vi "Core gRPC Server.vi"(8 "error in (no error)":errorcluster, 11 "CIFTemplateNode in":refnum<class "CIFCorePlugin.lvclass">) -> (0 "error out":errorcluster, 3 "CIFTemplateNode out":refnum<class "CIFCorePlugin.lvclass">)   [LabVIEW 2021, in "CIFCorePlugin.lvclass"]
uses:
  CIFCorePlugin.lvclass
  CIFCorePlugin.lvclass/CIFCorePlugin.ctl
  Grpc/CIFCorePlugin_server/RPC Service/PluginCore/PluginCore.lvclass
  Grpc/CIFCoreWrapper/CIFCoreWrapper.lvlib
  Grpc/CIFCorePlugin_client/RPC Messages/cif_common_Version.ctl
  Grpc/CIFCorePlugin_client/CIFCorePlugin_client.lvlib
  <vilib>/addons/_JKI.lib/Serialization/JSON/JKI JSON Serialization.lvlib
  Grpc/CIFCorePlugin_server/RPC Messages/cif_plugincore_Configuration.ctl
  Grpc/CIFCorePlugin_server/CIFCorePlugin_server.lvlib
  Grpc/CIFCorePlugin_server/RPC Messages/cif_plugincore_TimingOverrides.ctl
  Grpc/CIFCorePlugin_server/RPC Messages/cif_plugincore_PluginOverrides.ctl
  <vilib>/gRPC/LabVIEW gRPC Servicer/Servicer/Servicer.lvclass
  Common/CIFCoreCommon.lvlib
  Common/Typedef/Errors.ctl
  CIFUtilities/CIFLogs/CIFLogs.lvlib
  CIFUtilities/CIFLogs/Typedef/Plugin State Commands.ctl
  Grpc/CIFCoreChannel_server/RPC Service/ChannelCore/ChannelCore.lvclass
  Grpc/CIFCorePlugin_client/RPC Messages/cif_common_Status.ctl
  Grpc/CIFCoreChannel_server/RPC Messages/cif_channelcore_ChannelDirection.ctl
  Grpc/CIFCoreChannel_server/CIFCoreChannel_server.lvlib
  Grpc/CIFCoreChannel_server/RPC Messages/cif_channelcore_Channel.ctl
  Grpc/CIFCoreChannel_server/RPC Messages/cif_channelcore_Channels.ctl
  Grpc/CIFCorePlugin_client/RPC Messages/cif_common_PluginNames.ctl
  Common/Typedef/Channel Connection Data.ctl
  Common/Typedef/Channel Force Data.ctl
  Grpc/CIFCoreChannel_server/RPC Messages/cif_common_Status.ctl
  Grpc/CIFCoreChannel_server/RPC Messages/cif_channelcore_FIFOReference.ctl
  <vilib>/CIF Foundation/CIF Channels Core/ChannelCommon/typedef/New FIFO Instance Configuration.ctl
  <vilib>/CIF Foundation/CIF Channels Core/ChannelCommon/ChannelCommon.lvlib
  Common/Typedef/FIFO Publisher.ctl
  Channels/CIFChannelMng/CIFChannelMng.lvclass
  Grpc/CIFCoreChannel_server/RPC Messages/cif_channelcore_ChannelPattern.ctl
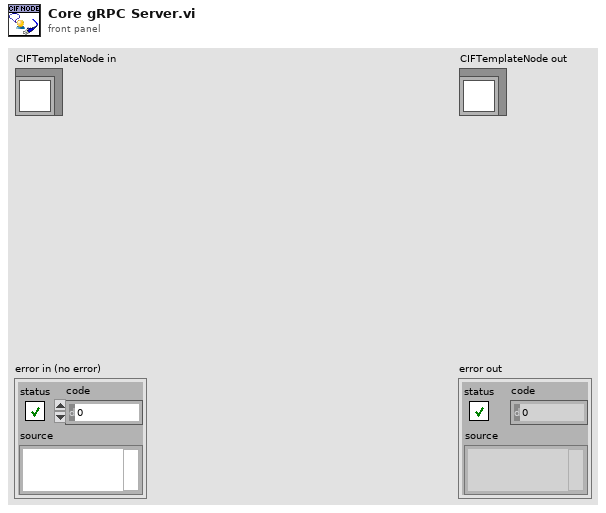
[diagram p1: front panel]
types:
  T1 = typedef "CIFCorePlugin_client.lvlib/cif_common_Status.ctl" = cluster{"code":i32, "message":string}
  T2 = typedef "CIFCorePlugin_client.lvlib/cif_common_PluginNames.ctl" = cluster{"plugin_name":string, "plugin_type":string}
  T3 = typedef "CIFCoreCommon.lvlib/Errors.ctl" = enum16{"Invalid Clock ID", "Long Sleep", "gRPC Server Not Found", "Config Parse", "Timestamp Wrap", "Delayed Execution", "Duplicate Channel", "Missing Channel", "Incorrect Type", "Flatten Error", "Unflatten Data", "Unique Name", "Plugin Not Found", "Plugin Type Not Found", "Plugin Version Not Found", "Manager Not Found", "Numerical Issue", "Time Jump", "Clock ID Match", "Channel Length", "Plugin Connection", "gRPC Server Connection", "PPL Name Match", "Build", "Config Log Parse", "Plugin Load", "UI Subpanel Load", "Python Name", "Invalid Name", "Unable to Change Ch Buffer"}
  T4 = typedef "CIFCorePlugin_client.lvlib/cif_common_Version.ctl" = cluster{"major":u32, "minor":u32, "fix":u32, "build":u32}
  T5 = typedef "CIFCorePlugin_server.lvlib/cif_plugincore_Configuration.ctl" = cluster{"json_config":string}
  T6 = typedef "CIFCorePlugin_server.lvlib/cif_plugincore_PluginOverrides.ctl" = cluster{"timing_overrides":T7}
  T7 = typedef "CIFCorePlugin_server.lvlib/cif_plugincore_TimingOverrides.ctl" = cluster{"override_timing":bool, "skip_sleep":bool, "period":dbl}
  T8 = typedef "CIFCoreCommon.lvlib/Channel Connection Data.ctl" = cluster{"Publisher Name":string, "Subscriber Name":string, "Connection Data":u8[]}
  T9 = typedef "CIFCoreCommon.lvlib/Channel Force Data.ctl" = cluster{"Channel Name":string, "Force Data":u8[], "Force Active":bool}
  T10 = typedef "CIFCoreCommon.lvlib/FIFO Publisher.ctl" = cluster{"Publisher Name":string, "New FIFO Instance Config":T11}
  T11 = typedef "ChannelCommon.lvlib/New FIFO Instance Configuration.ctl" = cluster{"Backpressure":bool, "Bytes/Message Override":u32, "Messages/FIFO Override":u32, "Custom Data":u8[]}
  T12 = typedef "CIFCoreChannel_server.lvlib/cif_channelcore_FIFOReference.ctl" = cluster{"publisher_instance_name":string, "custom_connect":u8[], "status":T13}
  T13 = typedef "CIFCoreChannel_server.lvlib/cif_common_Status.ctl" = cluster{"code":i32, "message":string}
  T14 = typedef "CIFCoreChannel_server.lvlib/cif_channelcore_Channels.ctl" = cluster{"channels":T15[]}
  T15 = typedef "CIFCoreChannel_server.lvlib/cif_channelcore_Channel.ctl" = cluster{"name":string, "direction":T16, "type":string, "custom_config":u8[], "connected":bool, "connected_name":string, "forced":bool, "channel_pattern":T17}
  T16 = typedef "CIFCoreChannel_server.lvlib/cif_channelcore_ChannelDirection.ctl" = enum32{"CHANNELDIRECTION_UNKNOWN", "CHANNELDIRECTION_PUBLISHER", "CHANNELDIRECTION_SUBSCRIBER"}
  T17 = typedef "CIFCoreChannel_server.lvlib/cif_channelcore_ChannelPattern.ctl" = enum32{"CHANNELPATTERN_UNKNOWN", "CHANNELPATTERN_TAG", "CHANNELPATTERN_FIFO", "CHANNELPATTERN_MULTIFIFO", "CHANNELPATTERN_BACKPRESSUREFIFO"}
  T18 = typedef "grpc-lvsupport-release.lvlib/grpcId.ctl" = u64
  T19 = typedef "CIFLogs.lvlib/Plugin State Commands.ctl" = enum16{"Create", "Configure", "Run", "Pause", "Destroy", "Connect", "Force", "FIFO Instance"}
  T20 = typedef "CIFCoreCommon.lvlib/Plugin Status.ctl" = cluster{"State":T21, "Timing Statistics (us)":T22, "FIFO Statistics (us)":T24, "error":T25, "Monitor Doubles":T26, "Monitor U64":T27, "Monitor I64":T28}
  T21 = typedef "CIFCoreCommon.lvlib/Plugin State.ctl" = enum32{"Null", "Creating", "Listening", "Running", "CleaningUp", "Destroying"}
  T22 = typedef "CIFCoreCommon.lvlib/Timing Statistics.ctl" = cluster{"Period":T23, "Wake Error":T23, "Execute":T23, "Housekeep":T23, "Idle":T23, "Cleanup":T23, "Custom 1":T23, "Custom 2":T23}
  T23 = typedef "CIFCoreCommon.lvlib/Timing Stats Base.ctl" = cluster{"Max":i64, "Avg":dbl, "Min":i64}
  T24 = typedef "CIFCoreCommon.lvlib/FIFO Statistics.ctl" = cluster{"From T0":T23, "From Previous Plugin":T23, "Output Error":T23}
  T25 = typedef "CIFCoreCommon.lvlib/Simple Error.ctl" = cluster{"status":bool, "code":i32}
  T26 = typedef "CIFCoreCommon.lvlib/Monitor Doubles.ctl" = cluster{"1":dbl, "2":dbl, "3":dbl, "4":dbl}
  T27 = typedef "CIFCoreCommon.lvlib/Monitor U64.ctl" = cluster{"1":u64, "2":u64, "3":u64, "4":u64}
  T28 = typedef "CIFCoreCommon.lvlib/Monitor I64.ctl" = cluster{"1":i64, "2":i64, "3":i64, "4":i64}
  T29 = typedef "CIFCorePlugin_client.lvlib/cif_plugincore_StatusData.ctl" = cluster{"state":T30, "timing_statistics":T31, "fifo_statistics":T33, "error":T34, "monitor_doubles":T35, "monitor_u64s":T36, "monitor_i64s":T37}
  T30 = typedef "CIFCorePlugin_client.lvlib/cif_plugincore_StatusData_PluginState.ctl" = enum32{"PLUGINSTATE_UNKNOWN", "PLUGINSTATE_CREATING", "PLUGINSTATE_LISTENING", "PLUGINSTATE_RUNNING", "PLUGINSTATE_CLEANINGUP", "PLUGINSTATE_DESTROYING"}
  T31 = typedef "CIFCorePlugin_client.lvlib/cif_plugincore_TimingStatistics.ctl" = cluster{"period":T32, "wake_error":T32, "execute":T32, "housekeep":T32, "idle":T32, "cleanup":T32, "custom_1":T32, "custom_2":T32}
  T32 = typedef "CIFCorePlugin_client.lvlib/cif_common_TimingStats.ctl" = cluster{"max":i64, "min":i64, "avg":dbl}
  T33 = typedef "CIFCorePlugin_client.lvlib/cif_plugincore_FifoStatistics.ctl" = cluster{"from_t0":T32, "from_previous_plugin":T32, "output_error":T32}
  T34 = typedef "CIFCorePlugin_client.lvlib/cif_plugincore_Error.ctl" = cluster{"status":bool, "code":i32}
  T35 = typedef "CIFCorePlugin_client.lvlib/cif_plugincore_MonitorDoubles.ctl" = cluster{"double_1":dbl, "double_2":dbl, "double_3":dbl, "double_4":dbl}
  T36 = typedef "CIFCorePlugin_client.lvlib/cif_plugincore_MonitorU64.ctl" = cluster{"u64_1":u64, "u64_2":u64, "u64_3":u64, "u64_4":u64}
  T37 = typedef "CIFCorePlugin_client.lvlib/cif_plugincore_MonitorI64.ctl" = cluster{"i64_1":i64, "i64_2":i64, "i64_3":i64, "i64_4":i64}
  T38 = typedef "CIFCoreCommon.lvlib/Version.ctl" = cluster{"Major":i32, "Minor":i32, "Fix":i32, "Build":i32}
  T39 = typedef "CIFCoreChannel_server.lvlib/cif_channelcore_ConnectSubscriber.ctl" = cluster{"subscriber_name":string, "publisher_name":string, "custom_connect":u8[]}
  T40 = typedef "CIFCoreChannel_server.lvlib/cif_channelcore_ForceChannel.ctl" = cluster{"channel_name":string, "force":bool, "force_data":u8[]}
  T41 = typedef "CIFCoreChannel_server.lvlib/cif_channelcore_FIFOInstance.ctl" = cluster{"publisher_name":string, "retry_on_timeout":bool, "bytes_per_message_override":u32, "message_per_fifo_override":u32, "custom_data":u8[]}
  T42 = typedef "CIFChannelMng.lvclass/FIFO Publisher Return.ctl" = cluster{"FIFO Instance Config":T43, "error":errorcluster, "Added":bool}
  T43 = typedef "ChannelCommon.lvlib/New FIFO Instance Response.ctl" = cluster{"Publisher":string, "Custom Data":u8[]}
  T44 = typedef "CIFCoreChannel_server.lvlib/cif_channelcore_FIFOInstanceName.ctl" = cluster{"publisher_instance_name":string}
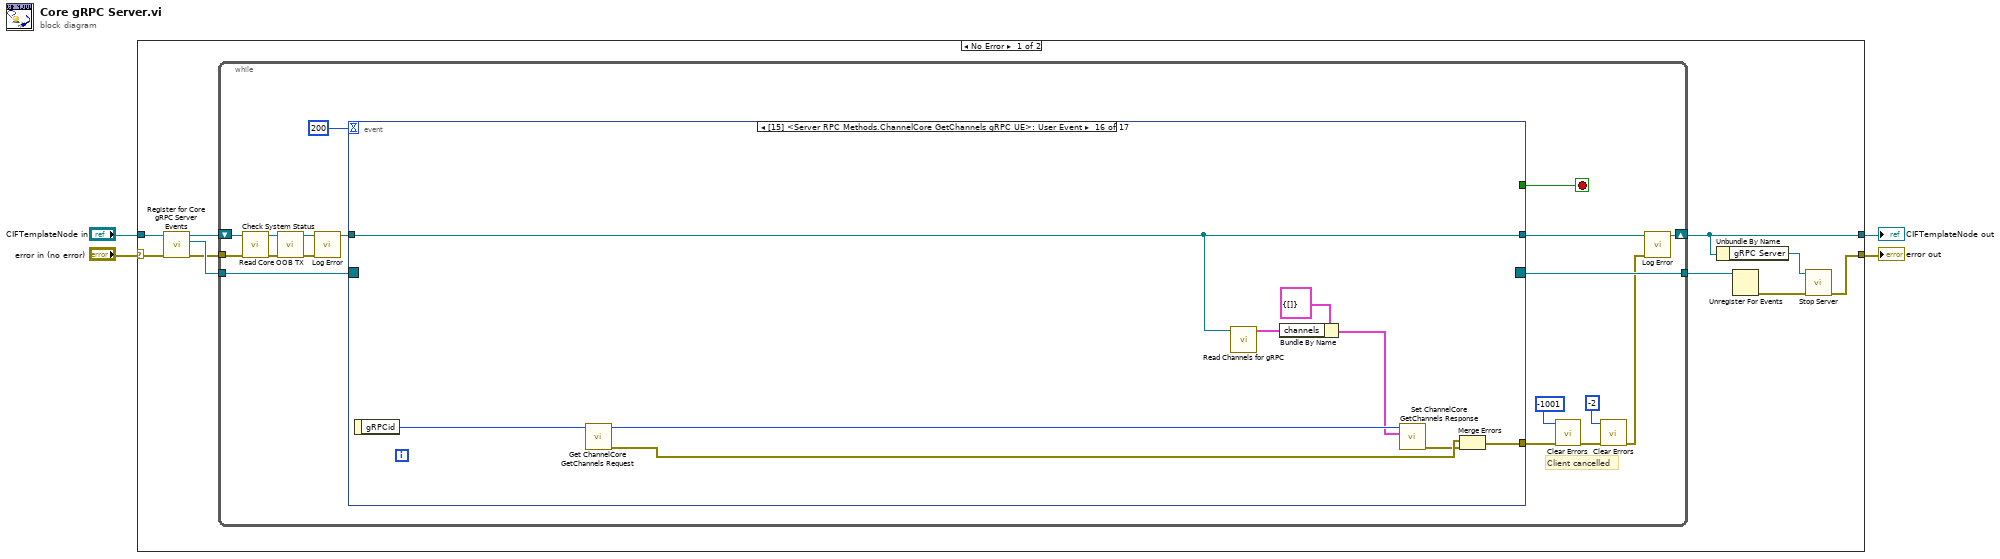
[diagram p0: block diagram]
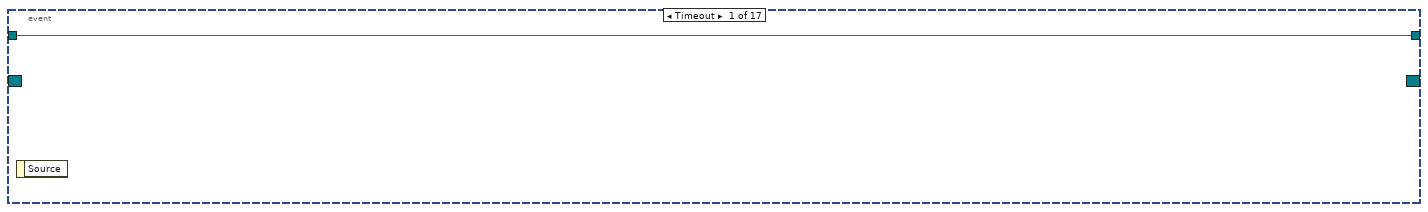
[diagram p2: hidden frame]
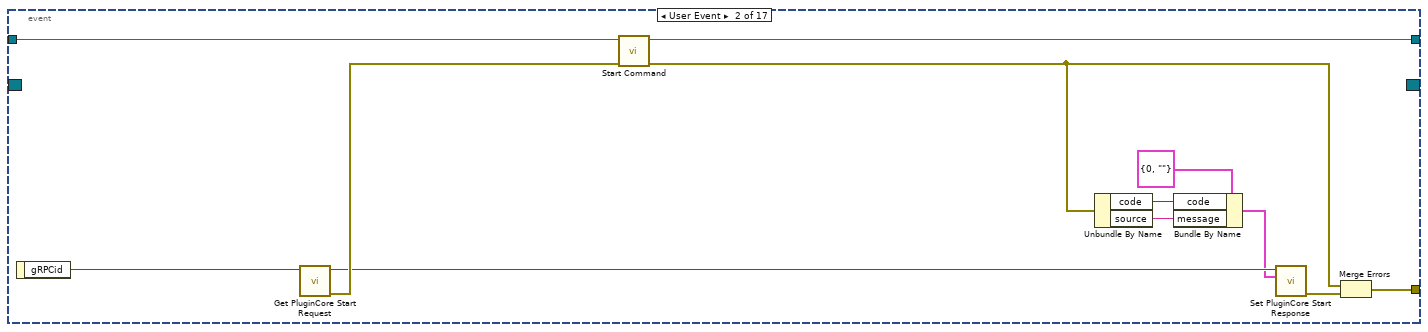
[diagram p3: hidden frame]
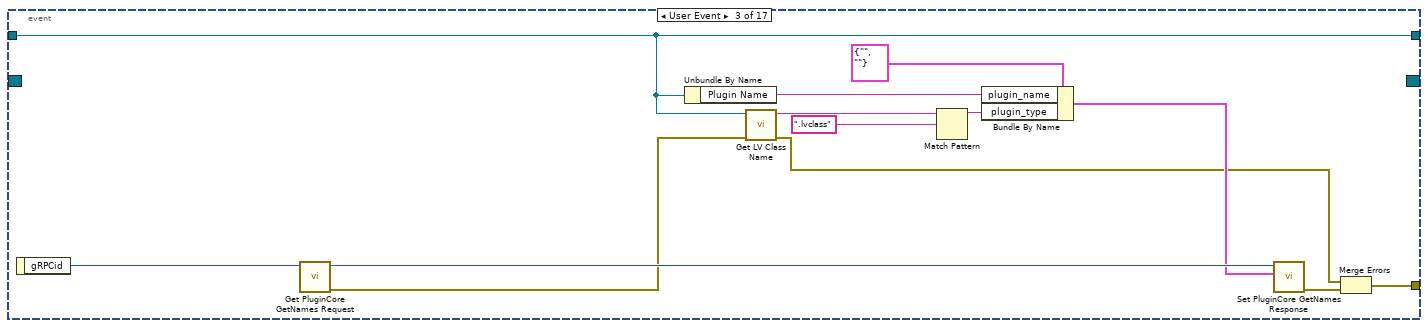
[diagram p4: hidden frame]
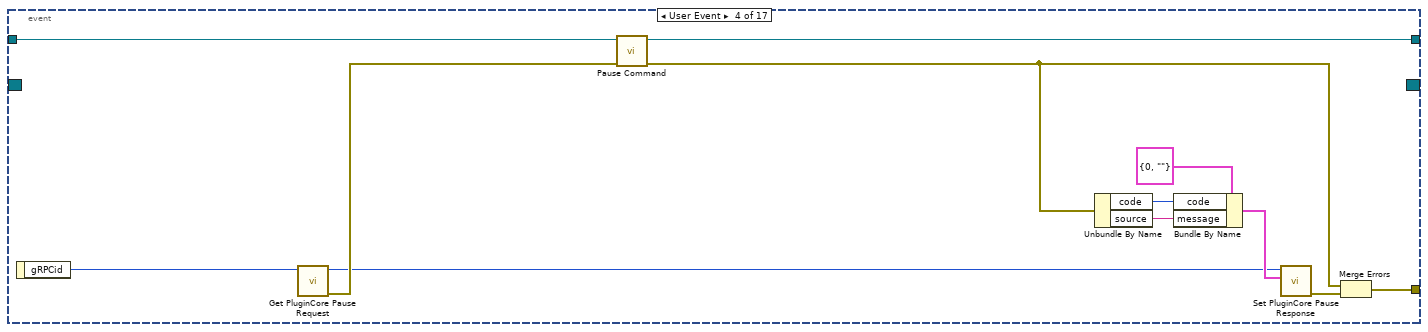
[diagram p5: hidden frame]
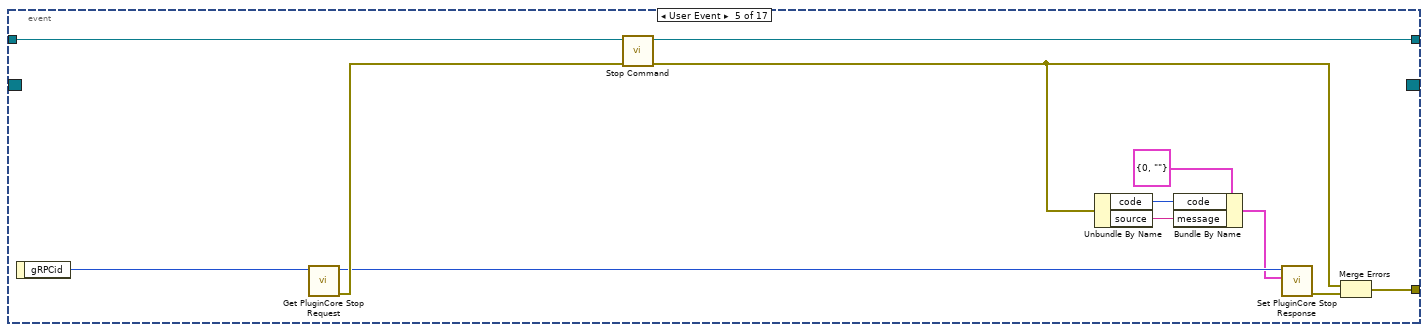
[diagram p6: hidden frame]
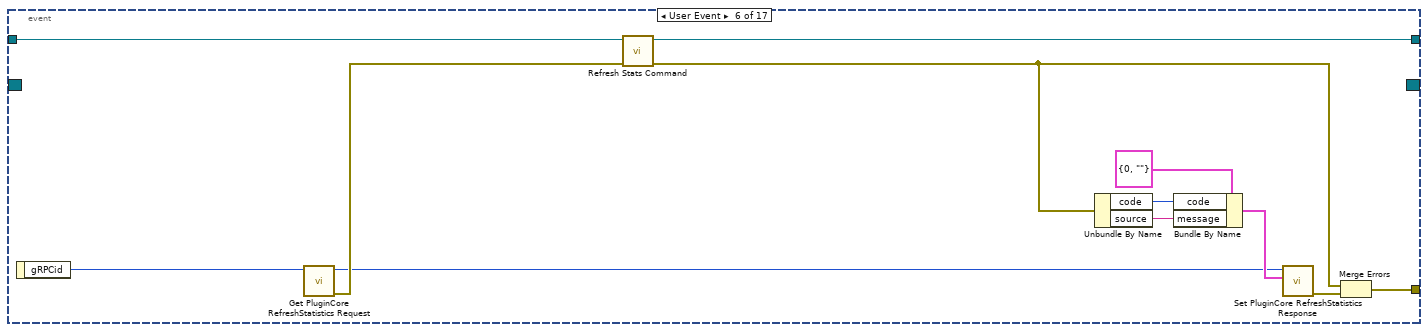
[diagram p7: hidden frame]
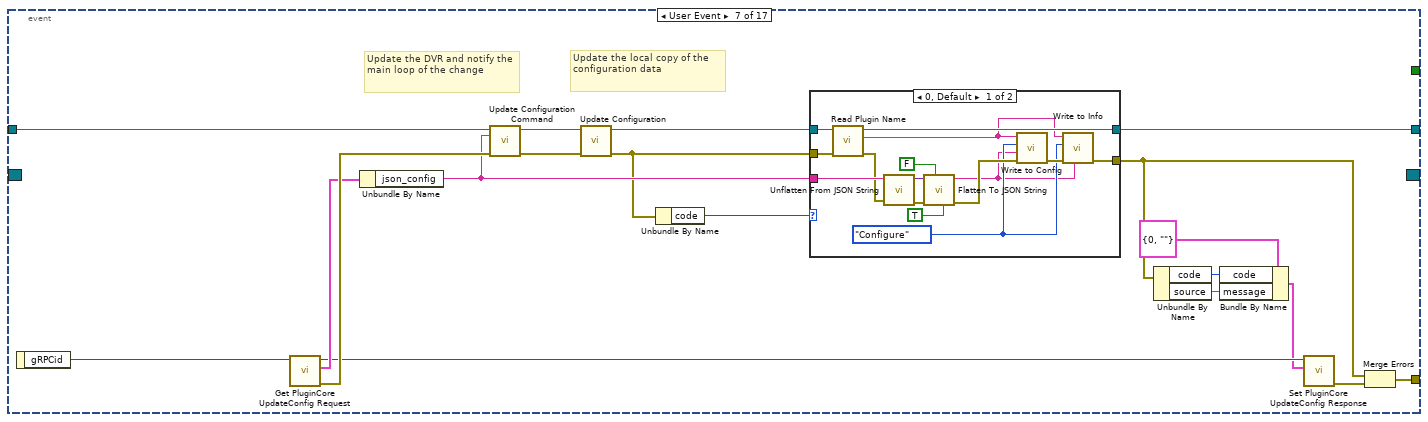
[diagram p8: hidden frame]
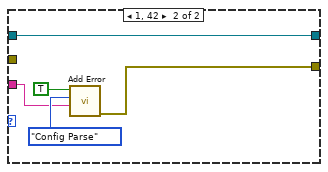
[diagram p9: hidden frame]
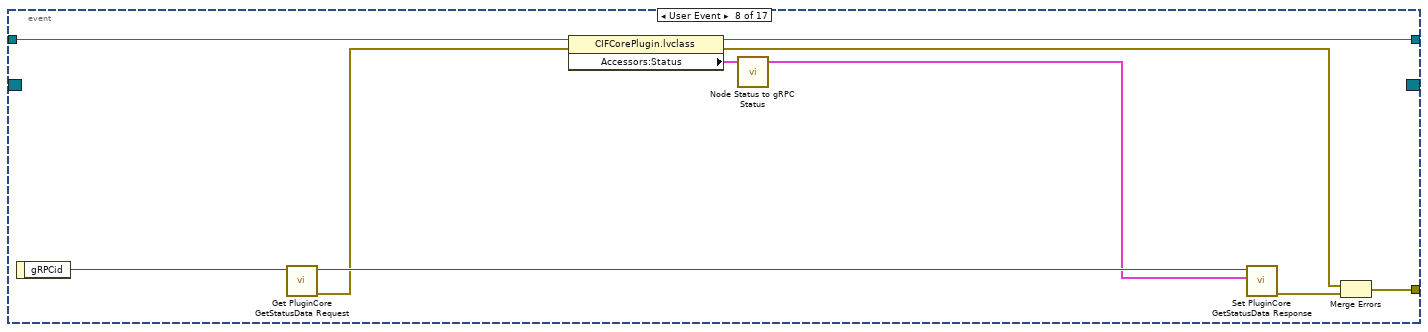
[diagram p10: hidden frame]
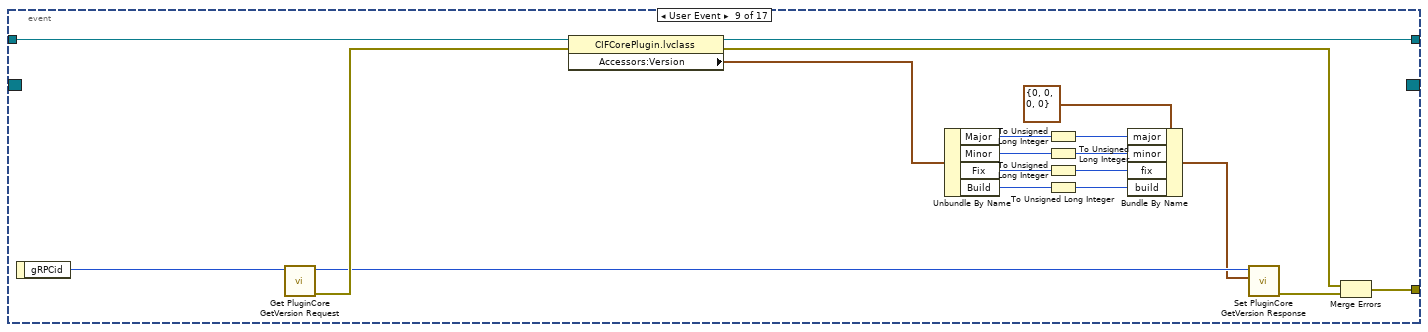
[diagram p11: hidden frame]
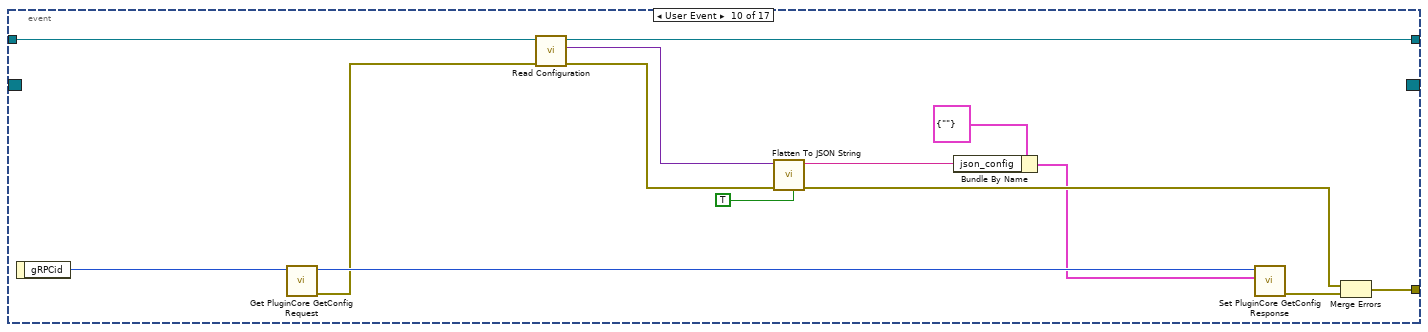
[diagram p12: hidden frame]
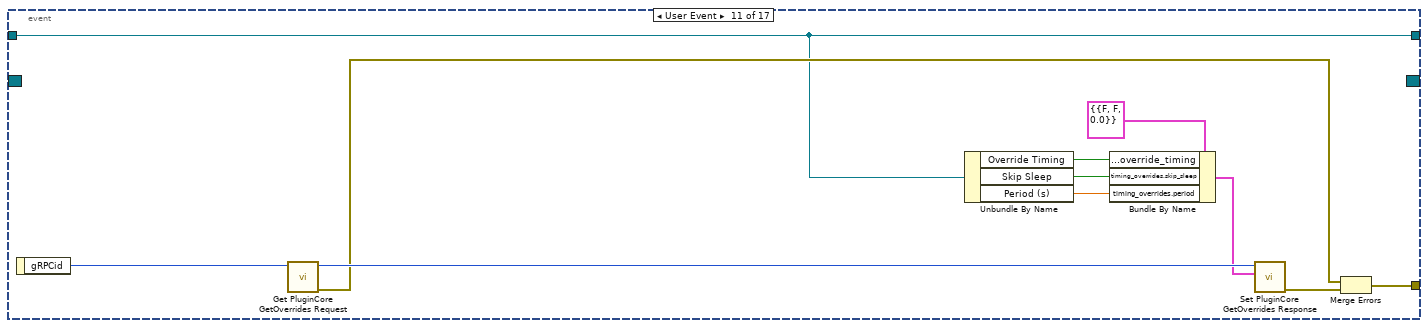
[diagram p13: hidden frame]
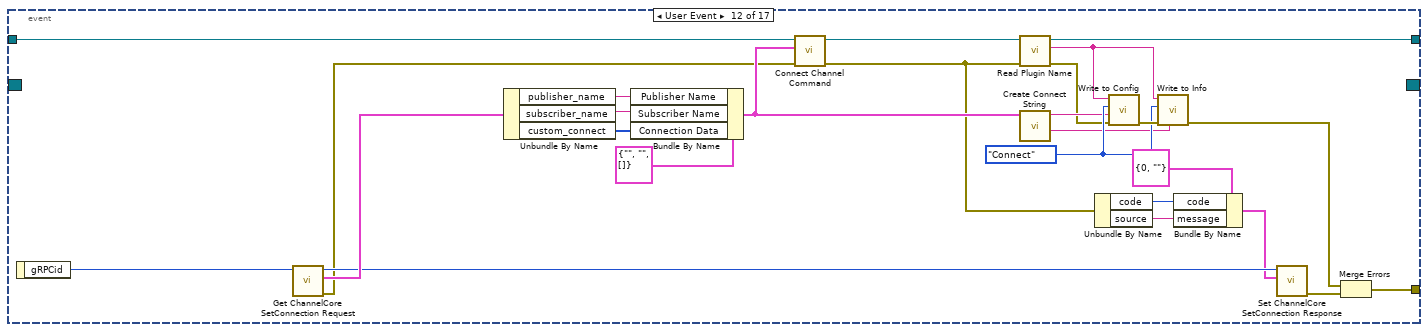
[diagram p14: hidden frame]
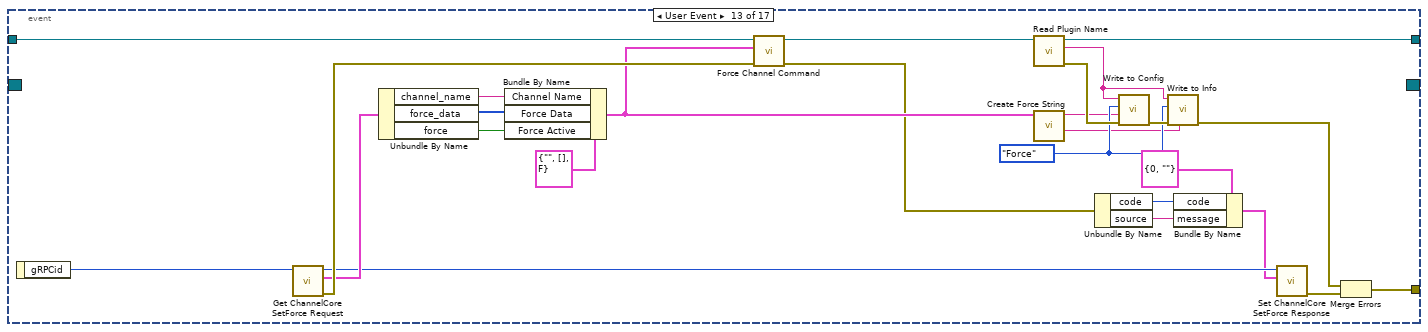
[diagram p15: hidden frame]
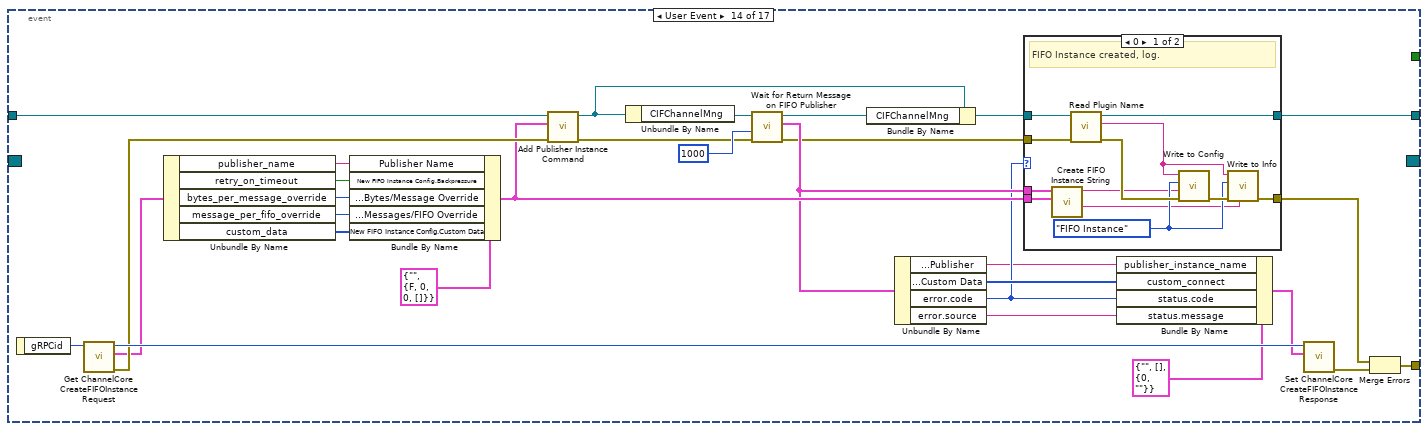
[diagram p16: hidden frame]
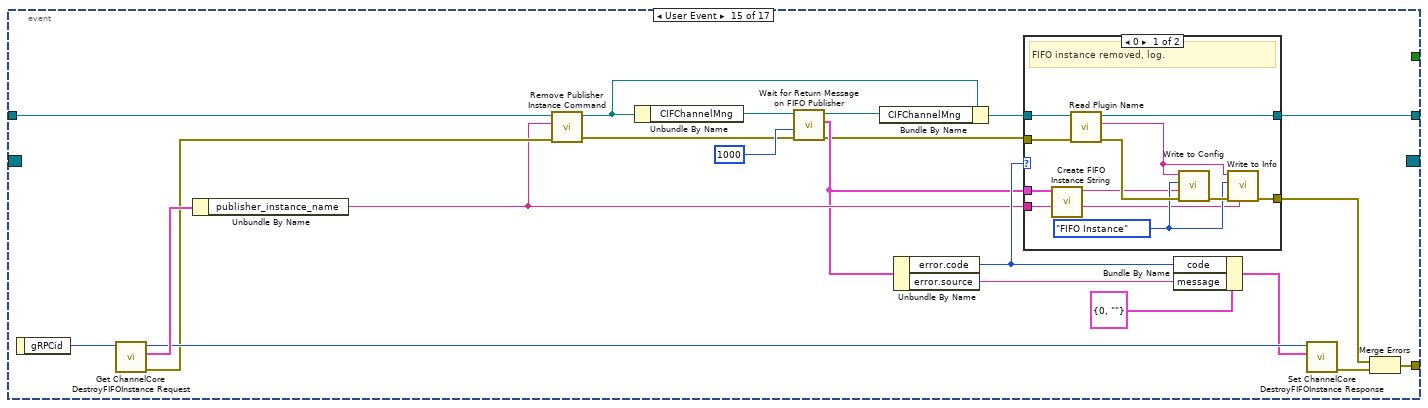
[diagram p18: hidden frame]
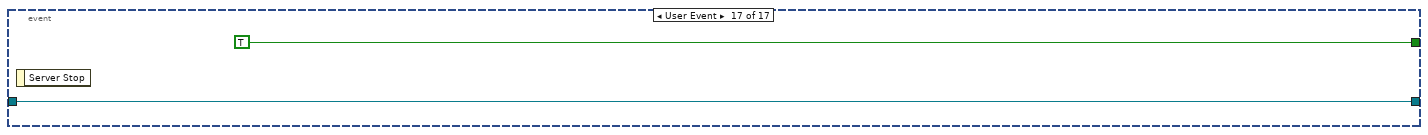
[diagram p20: hidden frame]
diagram:
  n1 = case shown="No Error" "error in (no error)" {
    selector: "error in (no error)" -> [w13 w331]
    tunnel: "CIFTemplateNode in" -> [w14 w332]
    tunnel: [w8 w332] -> w2
    tunnel: [w5 w331] -> w1
    frame No Error {
      n2 = call "Register for Core gRPC Server Events.vi"("error in (no error)"=w13, "CIFCorePlugin in"=w14) -> ("error out"=w11:errorcluster, "Event Registration Refnum"=w12:refnum<event-registration>, "CIFCorePlugin out"=w10:refnum<class "CIFCorePlugin.lvclass">)  [unwired: 7 in]
      n3 = while {
        tunnel: w12 -> [w32]
        tunnel: w11 -> [w23]
        tunnel: [w29] -> w9
        shift-right: [w27] -> w8
        shift-left: w10 -> [w22]
        stop <- w30 stop-if-true
        # "Client cancelled"
        n4 = call "Check System Status.vi"("error in (no error)"=w23, "CIFCorePlugin in"=w22) -> ("error out"=w21:errorcluster, "CIFCorePlugin out"=w20:refnum<class "CIFCorePlugin.lvclass">)  [unwired: 8 in]
        n5 = call "Read Core OOB TX.vi"("error in (no error)"=w21, "CIFCorePlugin in"=w20) -> ("error out"=w24:errorcluster, "CIFCorePlugin out"=w26:refnum<class "CIFCorePlugin.lvclass">)  [unwired: 8 in]
        n6 = call "Log Error.vi"("error in (no error)"=w24, "CIFCorePlugin in"=w26) -> ("CIFCorePlugin out"=w25:refnum<class "CIFCorePlugin.lvclass">)  [unwired: 8 in, 1 out]
        n7 = event shown="[15] <Server RPC Methods.ChannelCore GetChannels gRPC UE>: User Event" {
          selector: w32 -> [_ _ _ _ _ _ _ _ _ _ _ _ _ _ _ _ _]
          dyn-events: [_ _ _ _ _ _ _ _ _ _ _ _ _ _ _ _ _] -> w29
          timeout: 200 -> [_ _ _ _ _ _ _ _ _ _ _ _ _ _ _ _ _]
          tunnel: w25 -> [w33 w36 w52 w61 w73 w85 w100 w135 w161 w167 w180 w190 w215 w242 w287 w320 w329]
          tunnel: [_ w38 w57 w67 w79 w91 w113 w143 w162 w176 w187 w211 w237 w268 w304 w328 _] -> w18
          tunnel: [w33 w35 w52 w60 w72 w84 w101 w141 w160 w164 w180 w192 w218 w264 w303 w320 w329] -> w28
          tunnel: [_ _ _ _ _ _ _ _ _ _ _ _ _ _ _ _ TRUE] -> w30
          event Timeout {
            n8 = event-data() -> ()  [unwired: 1 in, 1 out]
          }
          event User Event {
            n9 = event-data() -> ("gRPCid"=w45:T18)  [unwired: 1 in]
            n10 = call "Get PluginCore Start Request.vi"("gRPCid"=w45) -> ("error out"=w44:errorcluster, "gRPCid out"=w43:T18)  [unwired: 8 in, 1 out]
            n11 = call "Start Command.vi"("error in"=w44, "CIFCorePlugin in"=w36) -> ("error out"=w34:errorcluster, "CIFCorePlugin out"=w35:refnum<class "CIFCorePlugin.lvclass">)  [unwired: 8 in]
            n12 = Unbundle By Name(w34) -> ("code"=w42:i32, "source"=w41:string)
            n13 = Bundle By Name(cluster=T1 {"code"=0, "message"=""} ("Message Data"), "code"=w42, "message"=w41) -> (w40:T1)
            n14 = call "Set PluginCore Start Response.vi"("Message Data"=w40, "gRPCid in"=w43) -> ("error out"=w39:errorcluster)  [unwired: 9 in]
            n15 = Merge Errors(w34, w39) -> (w38:errorcluster)
          }
          event User Event {
            n16 = event-data() -> ("gRPCid"=w56:T18)  [unwired: 1 in]
            n17 = call "Get PluginCore GetNames Request.vi"("gRPCid"=w56) -> ("error out"=w51:errorcluster, "gRPCid out"=w55:T18)  [unwired: 8 in, 1 out]
            n18 = Unbundle By Name(w52) -> ("Plugin Name"=w58:string)
            n19 = call <vilib>:"Get LV Class Name.vi"("error in (no error)"=w51, "object"=w52) -> ("error out"=w46:errorcluster, "class name"=w49:string)  [unwired: 8 in]
            n20 = Match Pattern(string=w49, regular expression=".lvclass") -> (before substring=w48:string)  [unwired: 1 in, 3 out]
            n21 = Bundle By Name(cluster=T2 {"plugin_name"="", "plugin_type"=""} ("Message Data"), "plugin_name"=w58, "plugin_type"=w48) -> (w50:T2)
            n22 = call "Set PluginCore GetNames Response.vi"("Message Data"=w50, "gRPCid in"=w55) -> ("error out"=w54:errorcluster)  [unwired: 9 in]
            n23 = Merge Errors(w46, w54) -> (w57:errorcluster)
          }
          event User Event {
            n24 = event-data() -> ("gRPCid"=w66:T18)  [unwired: 1 in]
            n25 = call "Get PluginCore Pause Request.vi"("gRPCid"=w66) -> ("error out"=w65:errorcluster, "gRPCid out"=w63:T18)  [unwired: 8 in, 1 out]
            n26 = call "Pause Command.vi"("error in"=w65, "CIFCorePlugin in"=w61) -> ("error out"=w59:errorcluster, "CIFCorePlugin out"=w60:refnum<class "CIFCorePlugin.lvclass">)  [unwired: 8 in]
            n27 = Unbundle By Name(w59) -> ("code"=w69:i32, "source"=w68:string)
            n28 = Bundle By Name(cluster=T1 {"code"=0, "message"=""} ("Message Data"), "code"=w69, "message"=w68) -> (w64:T1)
            n29 = call "Set PluginCore Pause Response.vi"("Message Data"=w64, "gRPCid in"=w63) -> ("error out"=w62:errorcluster)  [unwired: 9 in]
            n30 = Merge Errors(w59, w62) -> (w67:errorcluster)
          }
          event User Event {
            n31 = event-data() -> ("gRPCid"=w78:T18)  [unwired: 1 in]
            n32 = call "Get PluginCore Stop Request.vi"("gRPCid"=w78) -> ("error out"=w77:errorcluster, "gRPCid out"=w76:T18)  [unwired: 8 in, 1 out]
            n33 = call "Stop Command.vi"("error in"=w77, "CIFCorePlugin in"=w73) -> ("error out"=w71:errorcluster, "CIFCorePlugin out"=w72:refnum<class "CIFCorePlugin.lvclass">)  [unwired: 8 in]
            n34 = Unbundle By Name(w71) -> ("code"=w81:i32, "source"=w80:string)
            n35 = Bundle By Name(cluster=T1 {"code"=0, "message"=""} ("Message Data"), "code"=w81, "message"=w80) -> (w75:T1)
            n36 = call "Set PluginCore Stop Response.vi"("Message Data"=w75, "gRPCid in"=w76) -> ("error out"=w74:errorcluster)  [unwired: 9 in]
            n37 = Merge Errors(w71, w74) -> (w79:errorcluster)
          }
          event User Event {
            n38 = event-data() -> ("gRPCid"=w90:T18)  [unwired: 1 in]
            n39 = call "Get PluginCore RefreshStatistics Request.vi"("gRPCid"=w90) -> ("error out"=w89:errorcluster, "gRPCid out"=w86:T18)  [unwired: 8 in, 1 out]
            n40 = call "Refresh Stats Command.vi"("error in"=w89, "CIFCorePlugin in"=w85) -> ("error out"=w83:errorcluster, "CIFCorePlugin out"=w84:refnum<class "CIFCorePlugin.lvclass">)  [unwired: 8 in]
            n41 = Unbundle By Name(w83) -> ("code"=w93:i32, "source"=w92:string)
            n42 = Bundle By Name(cluster=T1 {"code"=0, "message"=""} ("Message Data"), "code"=w93, "message"=w92) -> (w88:T1)
            n43 = call "Set PluginCore RefreshStatistics Response.vi"("Message Data"=w88, "gRPCid in"=w86) -> ("error out"=w87:errorcluster)  [unwired: 9 in]
            n44 = Merge Errors(w83, w87) -> (w91:errorcluster)
          }
          event User Event {
            # "Update the local copy of the configuration data"
            # "Update the DVR and notify the main loop of the change"
            n45 = event-data() -> ("gRPCid"=w112:T18)  [unwired: 1 in]
            n46 = call "Get PluginCore UpdateConfig Request.vi"("gRPCid"=w112) -> ("error out"=w111:errorcluster, "Message Data"=w110:T5, "gRPCid out"=w108:T18)  [unwired: 8 in]
            n47 = Unbundle By Name(w110) -> ("json_config"=w106:string)
            n48 = call "Update Configuration Command.vi"("error in"=w111, "Config JSON"=w106, "CIFCorePlugin in"=w100) -> ("error out"=w97:errorcluster, "CIFCorePlugin out"=w98:refnum<class "CIFCorePlugin.lvclass">)  [unwired: 7 in]
            n49 = call-dynamic "Update Configuration.vi"("error in (no error)"=w97, "CIFTemplateNode in"=w98) -> ("error out"=w96:errorcluster, "CIFTemplateNode out"=w95:refnum<class "CIFCorePlugin.lvclass">)  [unwired: 8 in]
            n50 = Unbundle By Name(w96) -> ("code"=w107:i32)
            n51 = case shown="0, Default" w107 {
              tunnel: w96 -> [w127 _]
              tunnel: [w119 w132] -> w99
              tunnel: w106 -> [w124 w129]
              tunnel: w95 -> [w128 w133]
              tunnel: [w126 w133] -> w101
              frame 0, Default {
                w115 = Plugin_State_Commands."Configure" ("Command")
                n52 = call "Read Plugin Name.vi"("error in (no error)"=w127, "CIFTemplateNode in"=w128) -> ("error out"=w120:errorcluster, "Plugin Name"=w116:string, "CIFTemplateNode out"=w126:refnum<class "CIFCorePlugin.lvclass">)  [unwired: 7 in]
                n53 = call <vilib>:"Unflatten From JSON String.vi"("error in (no error)"=w120, "JSON String"=w124) -> ("error out"=w121:errorcluster, "Variant"=w125:variant)  [unwired: 8 in]
                n54 = call <vilib>:"Flatten To JSON String.vi"("Enums As String (F)"=TRUE, "Multiline (T)"=FALSE, "error in (no error)"=w121, "Variant"=w125) -> ("error out"=w118:errorcluster, "JSON String"=w114:string)  [unwired: 6 in]
                n55 = call "Write to Config.vi"("error in (no error)"=w118, "Additional Data"=w114, "Command"=w115, "Plugin Name"=w116) -> ("error out"=w117:errorcluster)  [unwired: 7 in]
                n56 = call "Write to Info.vi"("Additional Data"=w114, "error in (no error)"=w117, "Command"=w115, "Plugin Name"=w116) -> ("error out"=w119:errorcluster)  [unwired: 7 in]
              }
              frame 1, 42 {
                n57 = call "Add Error.vi"("String to Append"=w129, "Error"=Errors."Config Parse", "Insert Error"=TRUE) -> ("error out"=w132:errorcluster)  [unwired: 8 in]
              }
            }
            n58 = Unbundle By Name(w99) -> ("code"=w105:i32, "source"=w104:string)
            n59 = Bundle By Name(cluster=T1 {"code"=0, "message"=""} ("Message Data"), "code"=w105, "message"=w104) -> (w102:T1)
            n60 = call "Set PluginCore UpdateConfig Response.vi"("Message Data"=w102, "gRPCid in"=w108) -> ("error out"=w109:errorcluster)  [unwired: 9 in]
            n61 = Merge Errors(w99, w109) -> (w113:errorcluster)
          }
          event User Event {
            n62 = event-data() -> ("gRPCid"=w142:T18)  [unwired: 1 in]
            n63 = call "Get PluginCore GetStatusData Request.vi"("gRPCid"=w142) -> ("error out"=w137:errorcluster, "gRPCid out"=w138:T18)  [unwired: 8 in, 1 out]
            n64 = property class="CIFCorePlugin.lvclass"(reference=w135, error in=w137) -> (reference out=w141:refnum<class "CIFCorePlugin.lvclass">, error out=w136:errorcluster, "Accessors:Status"=w140:T20)
            n65 = call "Node Status to gRPC Status.vi"("Node Status"=w140) -> ("gRPC Status"=w134:T29)  [unwired: 3 in]
            n66 = call "Set PluginCore GetStatusData Response.vi"("Message Data"=w134, "gRPCid in"=w138) -> ("error out"=w139:errorcluster)  [unwired: 9 in]
            n67 = Merge Errors(w136, w139) -> (w143:errorcluster)
          }
          event User Event {
            n68 = event-data() -> ("gRPCid"=w158:T18)  [unwired: 1 in]
            n69 = call "Get PluginCore GetVersion Request.vi"("gRPCid"=w158) -> ("error out"=w157:errorcluster, "gRPCid out"=w156:T18)  [unwired: 8 in, 1 out]
            n70 = property class="CIFCorePlugin.lvclass"(reference=w161, error in=w157) -> (reference out=w160:refnum<class "CIFCorePlugin.lvclass">, error out=w159:errorcluster, "Accessors:Version"=w149:T38)
            n71 = Unbundle By Name(w149) -> ("Major"=w153:i32, "Minor"=w152:i32, "Fix"=w151:i32, "Build"=w150:i32)
            n72 = To Unsigned Long Integer(number=w153) -> (unsigned 32bit integer=w147:u32)
            n73 = To Unsigned Long Integer(number=w152) -> (unsigned 32bit integer=w146:u32)
            n74 = To Unsigned Long Integer(number=w151) -> (unsigned 32bit integer=w145:u32)
            n75 = To Unsigned Long Integer(number=w150) -> (unsigned 32bit integer=w144:u32)
            n76 = Bundle By Name(cluster=T4 {"major"=0, "minor"=0, "fix"=0, "build"=0} ("Message Data"), "major"=w147, "minor"=w146, "fix"=w145, "build"=w144) -> (w148:T4)
            n77 = call "Set PluginCore GetVersion Response.vi"("Message Data"=w148, "gRPCid in"=w156) -> ("error out"=w155:errorcluster)  [unwired: 9 in]
            n78 = Merge Errors(w159, w155) -> (w162:errorcluster)
          }
          event User Event {
            n79 = event-data() -> ("gRPCid"=w175:T18)  [unwired: 1 in]
            n80 = call "Get PluginCore GetConfig Request.vi"("gRPCid"=w175) -> ("error out"=w166:errorcluster, "gRPCid out"=w174:T18)  [unwired: 8 in, 1 out]
            n81 = call "Read Configuration.vi"("error in"=w166, "CIFCorePlugin in"=w167) -> ("error out"=w163:errorcluster, "Configuration Data"=w165:variant, "CIFCorePlugin out"=w164:refnum<class "CIFCorePlugin.lvclass">)  [unwired: 7 in]
            n82 = call <vilib>:"Flatten To JSON String.vi"("Enums As String (F)"=TRUE, "error in (no error)"=w163, "Variant"=w165) -> ("error out"=w171:errorcluster, "JSON String"=w170:string)  [unwired: 7 in]
            n83 = Bundle By Name(cluster=T5 {"json_config"=""} ("Message Data"), "json_config"=w170) -> (w169:T5)
            n84 = call "Set PluginCore GetConfig Response.vi"("Message Data"=w169, "gRPCid in"=w174) -> ("error out"=w173:errorcluster)  [unwired: 9 in]
            n85 = Merge Errors(w171, w173) -> (w176:errorcluster)
          }
          event User Event {
            n86 = event-data() -> ("gRPCid"=w186:T18)  [unwired: 1 in]
            n87 = call "Get PluginCore GetOverrides Request.vi"("gRPCid"=w186) -> ("error out"=w181:errorcluster, "gRPCid out"=w185:T18)  [unwired: 8 in, 1 out]
            n88 = Unbundle By Name(w180) -> ("Override Timing"=w179:bool, "Skip Sleep"=w177:bool, "Period (s)"=w178:dbl)
            n89 = Bundle By Name(cluster=T6 {"timing_overrides"={"override_timing"=FALSE, "skip_sleep"=FALSE, "period"=0.0}} ("Message Data"), "timing_overrides.override_timing"=w179, "timing_overrides.skip_sleep"=w177, "timing_overrides.period"=w178) -> (w182:T6)
            n90 = call "Set PluginCore GetOverrides Response.vi"("Message Data"=w182, "gRPCid in"=w185) -> ("error out"=w184:errorcluster)  [unwired: 9 in]
            n91 = Merge Errors(w181, w184) -> (w187:errorcluster)
          }
          event User Event {
            w199 = Plugin_State_Commands."Connect" ("Command")
            n92 = event-data() -> ("gRPCid"=w210:T18)  [unwired: 1 in]
            n93 = call "Get ChannelCore SetConnection Request.vi"("gRPCid"=w210) -> ("error out"=w196:errorcluster, "Message Data"=w209:T39, "gRPCid out"=w208:T18)  [unwired: 8 in]
            n94 = Unbundle By Name(w209) -> ("publisher_name"=w204:string, "subscriber_name"=w203:string, "custom_connect"=w202:u8[])
            n95 = Bundle By Name(cluster=T8 {"Publisher Name"="", "Subscriber Name"="", "Connection Data"=[]} ("Channel Connection Data"), "Publisher Name"=w204, "Subscriber Name"=w203, "Connection Data"=w202) -> (w198:T8)
            n96 = call "Connect Channel Command.vi"("error in"=w196, "Channel Connection Data"=w198, "CIFCorePlugin in"=w190) -> ("error out"=w188:errorcluster, "CIFCorePlugin out"=w189:refnum<class "CIFCorePlugin.lvclass">)  [unwired: 7 in]
            n97 = call "Read Plugin Name.vi"("error in (no error)"=w188, "CIFTemplateNode in"=w189) -> ("error out"=w195:errorcluster, "Plugin Name"=w200:string, "CIFTemplateNode out"=w192:refnum<class "CIFCorePlugin.lvclass">)  [unwired: 7 in]
            n98 = call "Create Connect String.vi"("Channel Connection Data"=w198) -> ("Connect info string"=w194:string, "Connect config string"=w197:string)  [unwired: 9 in]
            n99 = Unbundle By Name(w188) -> ("code"=w213:i32, "source"=w212:string)
            n100 = call "Write to Config.vi"("error in (no error)"=w195, "Additional Data"=w197, "Command"=w199, "Plugin Name"=w200) -> ("error out"=w201:errorcluster)  [unwired: 7 in]
            n101 = call "Write to Info.vi"("Additional Data"=w194, "error in (no error)"=w201, "Command"=w199, "Plugin Name"=w200) -> ("error out"=w191:errorcluster)  [unwired: 7 in]
            n102 = Bundle By Name(cluster=T1 {"code"=0, "message"=""} ("Message Data"), "code"=w213, "message"=w212) -> (w207:T1)
            n103 = call "Set ChannelCore SetConnection Response.vi"("Message Data"=w207, "gRPCid in"=w208) -> ("error out"=w206:errorcluster)  [unwired: 9 in]
            n104 = Merge Errors(w191, w206) -> (w211:errorcluster)
          }
          event User Event {
            w223 = Plugin_State_Commands."Force" ("Command")
            n105 = event-data() -> ("gRPCid"=w236:T18)  [unwired: 1 in]
            n106 = call "Get ChannelCore SetForce Request.vi"("gRPCid"=w236) -> ("error out"=w235:errorcluster, "Message Data"=w234:T40, "gRPCid out"=w233:T18)  [unwired: 8 in]
            n107 = Unbundle By Name(w234) -> ("channel_name"=w229:string, "force_data"=w228:u8[], "force"=w227:bool)
            n108 = Bundle By Name(cluster=T9 {"Channel Name"="", "Force Data"=[], "Force Active"=FALSE} ("Channel Force Data"), "Channel Name"=w229, "Force Data"=w228, "Force Active"=w227) -> (w222:T9)
            n109 = call "Force Channel Command.vi"("error in"=w235, "Channel Force Data"=w222, "CIFCorePlugin in"=w215) -> ("error out"=w216:errorcluster, "CIFCorePlugin out"=w214:refnum<class "CIFCorePlugin.lvclass">)  [unwired: 7 in]
            n110 = call "Read Plugin Name.vi"("CIFTemplateNode in"=w214) -> ("error out"=w226:errorcluster, "Plugin Name"=w225:string, "CIFTemplateNode out"=w218:refnum<class "CIFCorePlugin.lvclass">)  [unwired: 8 in]
            n111 = call "Create Force String.vi"("Channel Force Data"=w222) -> ("Force info string"=w220:string, "Force string"=w221:string)  [unwired: 9 in]
            n112 = Unbundle By Name(w216) -> ("code"=w239:i32, "source"=w238:string)
            n113 = call "Write to Config.vi"("error in (no error)"=w226, "Additional Data"=w221, "Command"=w223, "Plugin Name"=w225) -> ("error out"=w224:errorcluster)  [unwired: 7 in]
            n114 = call "Write to Info.vi"("Additional Data"=w220, "error in (no error)"=w224, "Command"=w223, "Plugin Name"=w225) -> ("error out"=w217:errorcluster)  [unwired: 7 in]
            n115 = Bundle By Name(cluster=T1 {"code"=0, "message"=""} ("Message Data"), "code"=w239, "message"=w238) -> (w232:T1)
            n116 = call "Set ChannelCore SetForce Response.vi"("Message Data"=w232, "gRPCid in"=w233) -> ("error out"=w231:errorcluster)  [unwired: 9 in]
            n117 = Merge Errors(w217, w231) -> (w237:errorcluster)
          }
          event User Event {
            n118 = event-data() -> ("gRPCid"=w262:T18)  [unwired: 1 in]
            n119 = call "Get ChannelCore CreateFIFOInstance Request.vi"("gRPCid"=w262) -> ("error out"=w259:errorcluster, "Message Data"=w258:T41, "gRPCid out"=w261:T18)  [unwired: 8 in]
            n120 = Unbundle By Name(w258) -> ("publisher_name"=w267:string, "retry_on_timeout"=w266:bool, "bytes_per_message_override"=w265:u32, "message_per_fifo_override"=w255:u32, "custom_data"=w241:u8[])
            n121 = Bundle By Name(cluster=T10 {"Publisher Name"="", "New FIFO Instance Config"={"Backpressure"=FALSE, "Bytes/Message Override"=0, "Messages/FIFO Override"=0, "Custom Data"=[]}} ("New FIFO Pub"), "Publisher Name"=w267, "New FIFO Instance Config.Backpressure"=w266, "New FIFO Instance Config.Bytes/Message Override"=w265, "New FIFO Instance Config.Messages/FIFO Override"=w255, "New FIFO Instance Config.Custom Data"=w241) -> (w253:T10)
            n122 = call "Add Publisher Instance Command.vi"("error in"=w259, "New Publisher"=w253, "CIFCorePlugin in"=w242) -> ("error out"=w243:errorcluster, "CIFCorePlugin out"=w244:refnum<class "CIFCorePlugin.lvclass">)  [unwired: 7 in]
            n123 = Unbundle By Name(w244) -> ("CIFChannelMng"=w248:refnum<class "CIFChannelMng.lvclass">)
            n124 = call "Wait for Return Message on FIFO Publisher.vi"("error in (no error)"=w243, "Timeout (ms)"=u32 1000, "CIFChannelMng in"=w248) -> ("error out"=w245:errorcluster, "FIFO Publisher"=w251:T42, "CIFChannelMng out"=w247:refnum<class "CIFChannelMng.lvclass">)  [unwired: 5 in, 1 out]
            n125 = Bundle By Name(cluster=w244, "CIFChannelMng"=w247) -> (w249:refnum<class "CIFCorePlugin.lvclass">)
            n126 = Unbundle By Name(w251) -> ("FIFO Instance Config.Publisher"=w240:string, "FIFO Instance Config.Custom Data"=w254:u8[], "error.code"=w250:i32, "error.source"=w269:string)
            n127 = case shown="0" w250 {
              tunnel: w249 -> [w277 w283]
              tunnel: [w276 w283] -> w264
              tunnel: [w275 w282] -> w263
              tunnel: w245 -> [w274 w282]
              tunnel: w253 -> [w271 _]
              tunnel: w251 -> [w270 _]
              frame 0 {
                w278 = Plugin_State_Commands."FIFO Instance" ("Command")
                # "FIFO Instance created, log."
                n128 = call "Create FIFO Instance String.vi"("New FIFO Pub"=w271, "FIFO Publisher"=w270) -> ("FIFO Instance info string"=w272:string, "FIFO Instance string"=w273:string)  [unwired: 8 in]
                n129 = call "Read Plugin Name.vi"("error in (no error)"=w274, "CIFTemplateNode in"=w277) -> ("error out"=w281:errorcluster, "Plugin Name"=w280:string, "CIFTemplateNode out"=w276:refnum<class "CIFCorePlugin.lvclass">)  [unwired: 7 in]
                n130 = call "Write to Config.vi"("error in (no error)"=w281, "Additional Data"=w273, "Command"=w278, "Plugin Name"=w280) -> ("error out"=w279:errorcluster)  [unwired: 7 in]
                n131 = call "Write to Info.vi"("Additional Data"=w272, "error in (no error)"=w279, "Command"=w278, "Plugin Name"=w280) -> ("error out"=w275:errorcluster)  [unwired: 7 in]
              }
              frame 1, Default {
                # "Error or warning, FIFO instance not created, don't log."
              }
            }
            n132 = Bundle By Name(cluster=T12 {"publisher_instance_name"="", "custom_connect"=[], "status"={"code"=0, "message"=""}} ("Message Data"), "publisher_instance_name"=w240, "custom_connect"=w254, "status.code"=w250, "status.message"=w269) -> (w252:T12)
            n133 = call "Set ChannelCore CreateFIFOInstance Response.vi"("Message Data"=w252, "gRPCid in"=w261) -> ("error out"=w260:errorcluster)  [unwired: 9 in]
            n134 = Merge Errors(w263, w260) -> (w268:errorcluster)
          }
          event User Event {
            n135 = event-data() -> ("gRPCid"=w300:T18)  [unwired: 1 in]
            n136 = call "Get ChannelCore DestroyFIFOInstance Request.vi"("gRPCid"=w300) -> ("error out"=w294:errorcluster, "Message Data"=w299:T44, "gRPCid out"=w298:T18)  [unwired: 8 in]
            n137 = Unbundle By Name(w299) -> ("publisher_instance_name"=w293:string)
            n138 = call "Remove Publisher Instance Command.vi"("error in"=w294, "Publisher Name"=w293, "CIFCorePlugin in"=w287) -> ("error out"=w284:errorcluster, "CIFCorePlugin out"=w286:refnum<class "CIFCorePlugin.lvclass">)  [unwired: 7 in]
            n139 = Unbundle By Name(w286) -> ("CIFChannelMng"=w291:refnum<class "CIFChannelMng.lvclass">)
            n140 = call "Wait for Return Message on FIFO Publisher.vi"("error in (no error)"=w284, "Timeout (ms)"=u32 1000, "CIFChannelMng in"=w291) -> ("error out"=w285:errorcluster, "FIFO Publisher"=w292:T42, "CIFChannelMng out"=w290:refnum<class "CIFChannelMng.lvclass">)  [unwired: 5 in, 1 out]
            n141 = Bundle By Name(cluster=w286, "CIFChannelMng"=w290) -> (w288:refnum<class "CIFCorePlugin.lvclass">)
            n142 = Unbundle By Name(w292) -> ("error.code"=w301:i32, "error.source"=w305:string)
            n143 = case shown="0" w301 {
              tunnel: w288 -> [w313 w319]
              tunnel: [w312 w319] -> w303
              tunnel: [w311 w318] -> w302
              tunnel: w285 -> [w310 w318]
              tunnel: w292 -> [w307 _]
              tunnel: w293 -> [w306 _]
              frame 0 {
                w314 = Plugin_State_Commands."FIFO Instance" ("Command")
                # "FIFO instance removed, log."
                n144 = call "Create FIFO Instance String.vi"("Removal Channel"=w306, "FIFO Publisher"=w307) -> ("FIFO Instance info string"=w308:string, "FIFO Instance string"=w309:string)  [unwired: 8 in]
                n145 = call "Read Plugin Name.vi"("error in (no error)"=w310, "CIFTemplateNode in"=w313) -> ("error out"=w317:errorcluster, "Plugin Name"=w316:string, "CIFTemplateNode out"=w312:refnum<class "CIFCorePlugin.lvclass">)  [unwired: 7 in]
                n146 = call "Write to Config.vi"("error in (no error)"=w317, "Additional Data"=w309, "Command"=w314, "Plugin Name"=w316) -> ("error out"=w315:errorcluster)  [unwired: 7 in]
                n147 = call "Write to Info.vi"("Additional Data"=w308, "error in (no error)"=w315, "Command"=w314, "Plugin Name"=w316) -> ("error out"=w311:errorcluster)  [unwired: 7 in]
              }
              frame 1, Default {
                # "Error or warning, FIFO instance not removed, don't log."
              }
            }
            n148 = Bundle By Name(cluster=T13 {"code"=0, "message"=""} ("Message Data"), "code"=w301, "message"=w305) -> (w295:T13)
            n149 = call "Set ChannelCore DestroyFIFOInstance Response.vi"("Message Data"=w295, "gRPCid in"=w298) -> ("error out"=w297:errorcluster)  [unwired: 9 in]
            n150 = Merge Errors(w302, w297) -> (w304:errorcluster)
          }
          event User Event {
            n151 = event-data() -> ("gRPCid"=w327:T18)  [unwired: 1 in]
            n152 = call "Get ChannelCore GetChannels Request.vi"("gRPCid"=w327) -> ("error out"=w326:errorcluster, "gRPCid out"=w325:T18)  [unwired: 8 in, 1 out]
            n153 = call "Read Channels for gRPC.vi"("CIFCorePlugin in"=w320) -> ("Channels"=w321:T15[])  [unwired: 10 in]
            n154 = Bundle By Name(cluster=T14 {"channels"=[]} ("Message Data"), "channels"=w321) -> (w323:T14)
            n155 = call "Set ChannelCore GetChannels Response.vi"("Message Data"=w323, "gRPCid in"=w325) -> ("error out"=w322:errorcluster)  [unwired: 9 in]
            n156 = Merge Errors(w326, w322) -> (w328:errorcluster)
          }
          event User Event {
            n157 = event-data() -> ()  [unwired: 1 in, 1 out]
          }
        }
        n158 = call <vilib>:"Clear Errors.vi"("error in (no error)"=w18, "specific error code to clear (0: all)"=-1001) -> ("error out"=w17:errorcluster)  [unwired: 4 in, 1 out]
        n159 = call <vilib>:"Clear Errors.vi"("error in (no error)"=w17, "specific error code to clear (0: all)"=-2) -> ("error out"=w16:errorcluster)  [unwired: 4 in, 1 out]
        n160 = call "Log Error.vi"("error in (no error)"=w16, "CIFCorePlugin in"=w28) -> ("CIFCorePlugin out"=w27:refnum<class "CIFCorePlugin.lvclass">)  [unwired: 8 in, 1 out]
      }
      n161 = Unbundle By Name(w8) -> ("gRPC Server"=w7:refnum<class "Servicer.lvclass">)
      n162 = Unregister For Events(event registration refnum=w9) -> (error out=w6:errorcluster)  [unwired: 1 in]
      n163 = call <vilib>:"Stop Server.vi"("error in"=w6, "gRPC Server in"=w7) -> ("error out"=w5:errorcluster)  [unwired: 9 in]
    }
    frame Error {
    }
  }
  "error out" <- w1
  "CIFTemplateNode out" <- w2
